vi "Station_NG Station.vi"(8 "error in (no error)":errorcluster, 11 "Main":T1={"Tite"="", "Base path"=path "", "Table"=[], "Stations"=[], "Shield Array"=[], "UPHs"=[], "VISA"={"VISA"="", "baud rate"=9600, "data bits"=8, "parity"=enum."None", "stop bits"=10, "flow control"=0}, "Path"={"roof"=path "", "Config"=path "", "Png"=path ""}, "Ctr"={"DB Dispaly"=refnum, "Error Table"=refnum, "Display"=refnum, "Login"=refnum, "Exit"=refnum, "FTT_Submit"=refnum}, "Login"={"User"="", "Grade"=""}, "information"={"cause"="", "Type"=enum."Inform", "code"=0, "Suroce"="", "Status"=FALSE}, "Local DB"={"Connstr"="", "Database"={"Constr"={"Driver"="", "Server"="", "User"="", "Pwd"="", "Database"=""}, "conn ref"=refnum, "State"=FALSE}}, "Remote DB"={"Connstr"="", "Database"={"Constr"={"Driver"="", "Server"="", "User"="", "Pwd"="", "Database"=""}, "conn ref"=refnum, "State"=FALSE}}, "FTT TV"="", "ExchangeTime"=0, "NVH"="", "EOL Path"=path ""} {"VISA"."flow control" items=["None", "XON/XOFF", "RTS/CTS", "XON/XOFF & RTS/CTS", "DTR/DSR", "XON/XOFF & DTR/DSR"]; "VISA"."stop bits" items=["1.0"=10, "1.5"=15, "2.0"=20]}) -> (0 "error out":errorcluster)   [LabVIEW 2014]
uses:
  Type'def/Online_Table.ctl
  <vilib>/addons/database/_DB Variant To Data/Database Variant To Data.xnode
  Simatic S7/Function/Read/Read Sigle Data/Read Sigle String.vi
  Simatic S7/Function/Read/Read Sigle Data/Read Sigle Word.vi
  Type'def/UPH Config.ctl
  VISA/Ctr/VISA Ctr.ctl
  Type'def/Main Ctr Ref.ctl
  Type'def/User Login.ctl
  Database/Ctr/Constr.ctl
  <vilib>/addons/database/Connection.llb/Conn ObjectReference.ctl
  <vilib>/addons/database/NI_Database_API.lvlib
  Database/Ctr/Conneect State.ctl
  Type'def/MainCtr.ctl
panel:
  in  "t":u16
  in  "s":bool
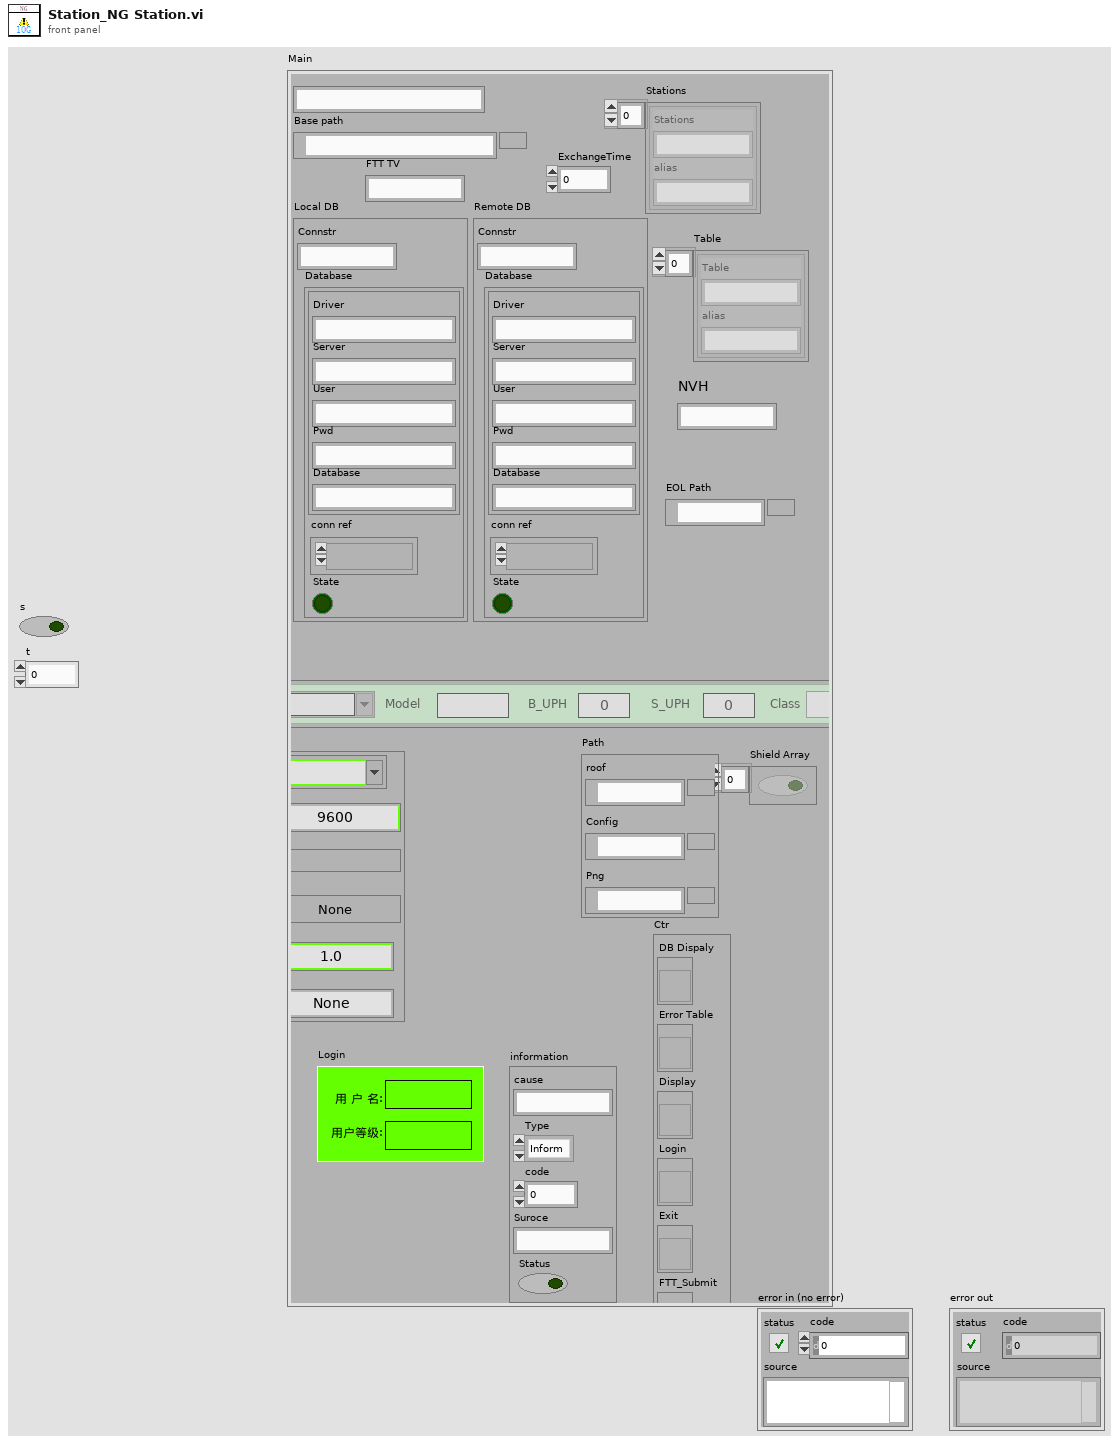
[diagram p1: front panel]
types:
  T1 = typedef "MainCtr.ctl" = cluster{"Tite":string, "Base path":path, "Table":cluster{"Table":string, "alias":string}[], "Stations":cluster{"Stations":string, "alias":string}[], "Shield Array":bool[], "UPHs":T2[], "VISA":T3, "Path":cluster{"roof":path, "Config":path, "Png":path}, "Ctr":T4, "Login":T5, "information":cluster{"cause":string, "Type":enum16{"Inform", "Warning", "Alarm"}, "code":i32, "Suroce":string, "Status":bool}, "Local DB":cluster{"Connstr":string, "Database":T6}, "Remote DB":cluster{"Connstr":string, "Database":T6}, "FTT TV":string, "ExchangeTime":i32, "NVH":string, "EOL Path":path}
  T2 = typedef "UPH Config.ctl" = cluster{"Line_No":string, "Model":string, "B_UPH ":i16, "S_UPH  ":i16, "Class":enum16{"Big", "Small"}}
  T3 = typedef "VISA Ctr.ctl" = cluster{"VISA":refnum<visa-resource-name>, "baud rate":u32, "data bits":u16, "parity":enum16{"None", "Odd", "Even", "Mark", "Space"}, "stop bits":u16, "flow control":u16}
  T4 = typedef "Main Ctr Ref.ctl" = cluster{"DB Dispaly":refnum<vi>, "Error Table":refnum<vi>, "Display":refnum<vi>, "Login":refnum<vi>, "Exit":refnum<vi>, "FTT_Submit":refnum<vi>}
  T5 = typedef "User Login.ctl" = cluster{"User":string, "Grade":string}
  T6 = typedef "Conneect State.ctl" = cluster{"Constr":T7, "conn ref":T8, "State":bool}
  T7 = typedef "Constr.ctl" = cluster{"Driver":string, "Server":string, "User":string, "Pwd":string, "Database":string}
  T8 = typedef "NI_Database_API.lvlib/Conn ObjectReference.ctl" = refnum<k1>
  T9 = cluster{"cause":string, "Type":enum16{"Inform", "Warning", "Alarm"}, "code":i32, "Suroce":string, "Status":bool}
  T10 = typedef "Online_Table.ctl" = cluster{"SN":string, "Frame":string, "Station":string, "Model":string, "Color":string, "OnTime":timestamp, "OutTime":timestamp, "Repaired":i32, "OnRepair":bool, "Pstate":string}
  T11 = cluster{"Main ":T1, "Online_Table":T10, "information":cluster{"cause":string, "Type":enum16{"Inform", "Warning", "Alarm"}, "code":i32, "Suroce":string, "Status":bool}, "Previous ":u16, "Station pos":i32[], "Pos":i32}
  T12 = typedef "FTT Display Type.ctl" = cluster{"Line.No":string, "Model":string, "Color":string, "UPH":dbl, "Plan":dbl, "Target Rate":dbl, "Target ":dbl, "Actual":dbl, "FTT":dbl, "FTT Rate":dbl, "Repaired":dbl, "Reject":dbl, "Ouline":dbl, "Line State":string}
  T13 = cluster{"Display":T12, "Class":enum16{"Big", "Small"}}
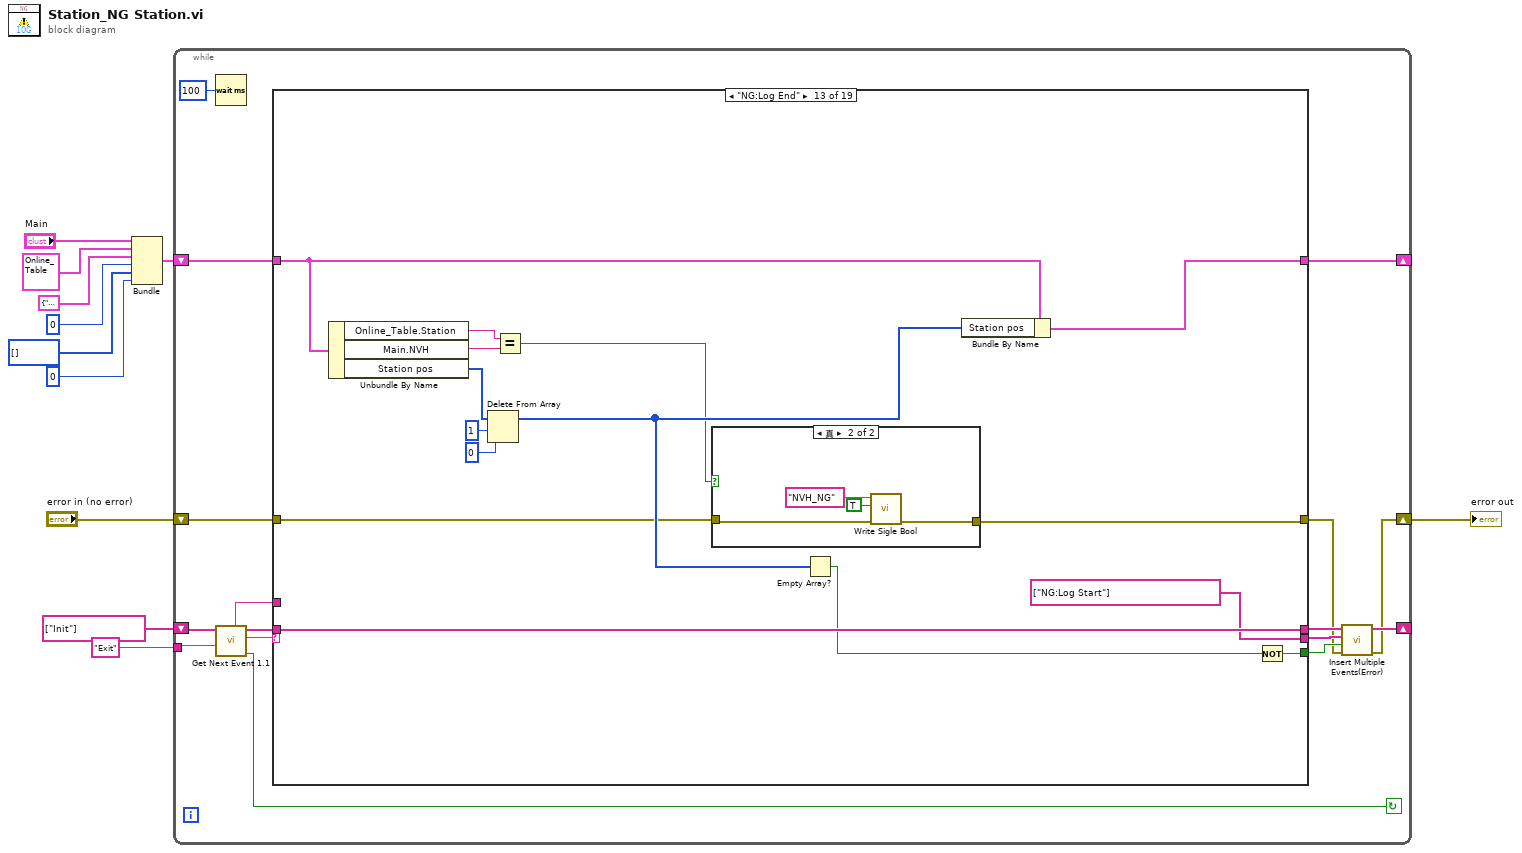
[diagram p0: block diagram]
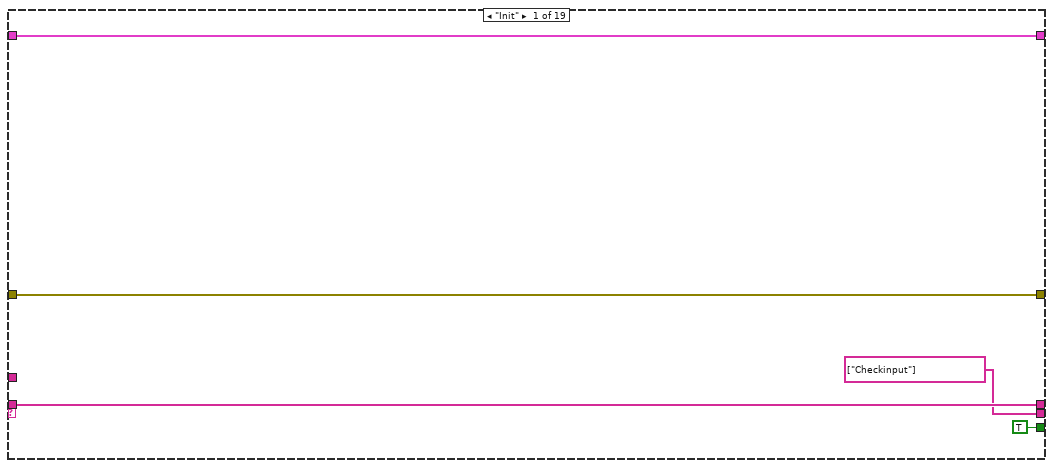
[diagram p2: hidden frame]
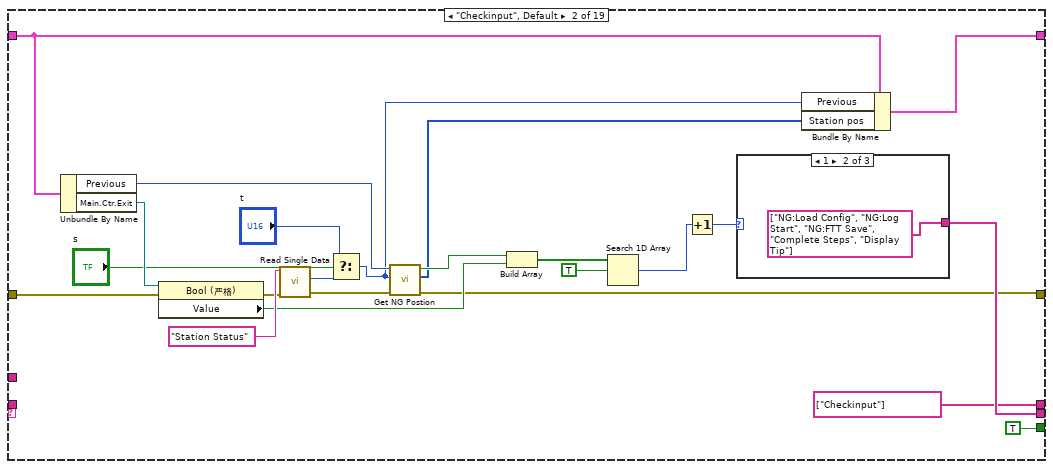
[diagram p3: hidden frame]
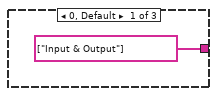
[diagram p4: hidden frame]
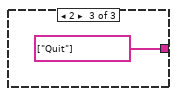
[diagram p5: hidden frame]
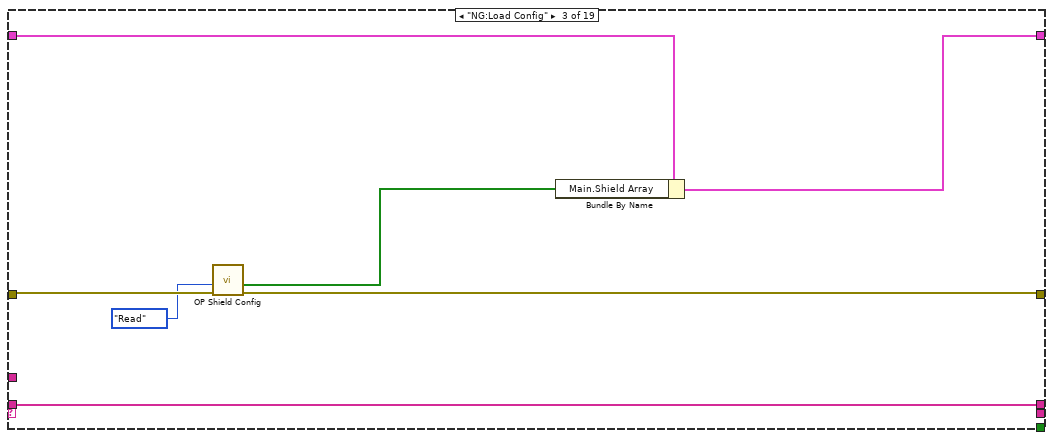
[diagram p6: hidden frame]
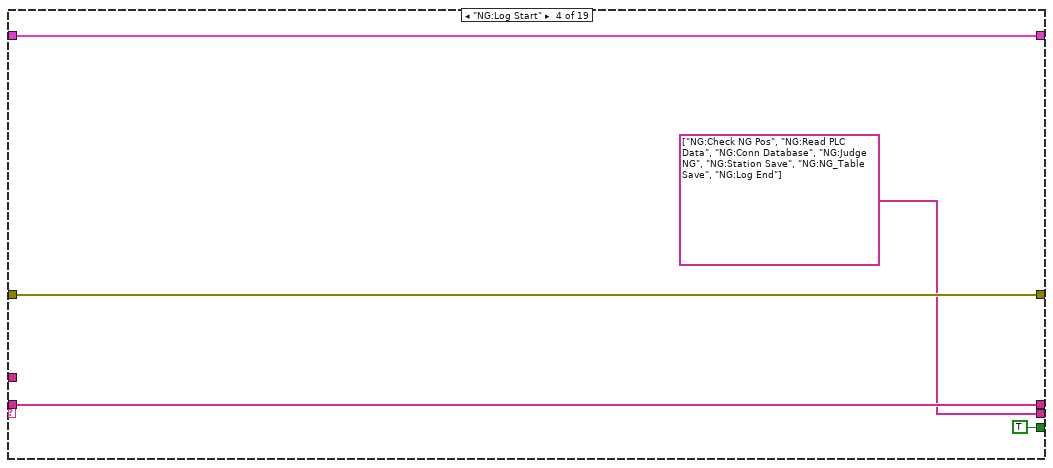
[diagram p7: hidden frame]
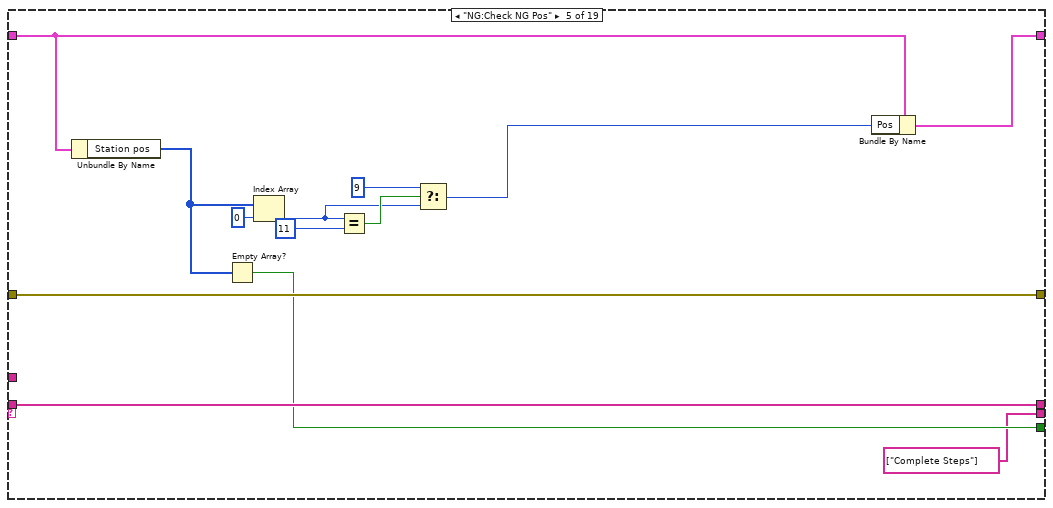
[diagram p8: hidden frame]
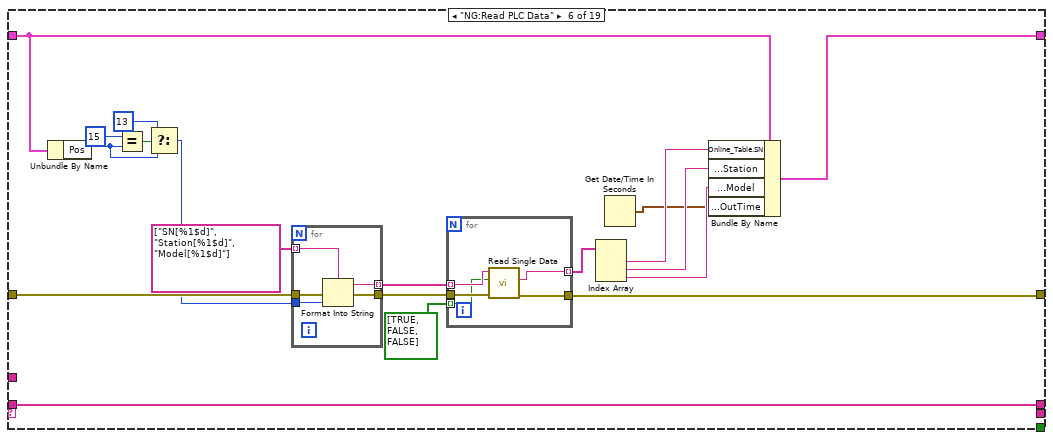
[diagram p9: hidden frame]
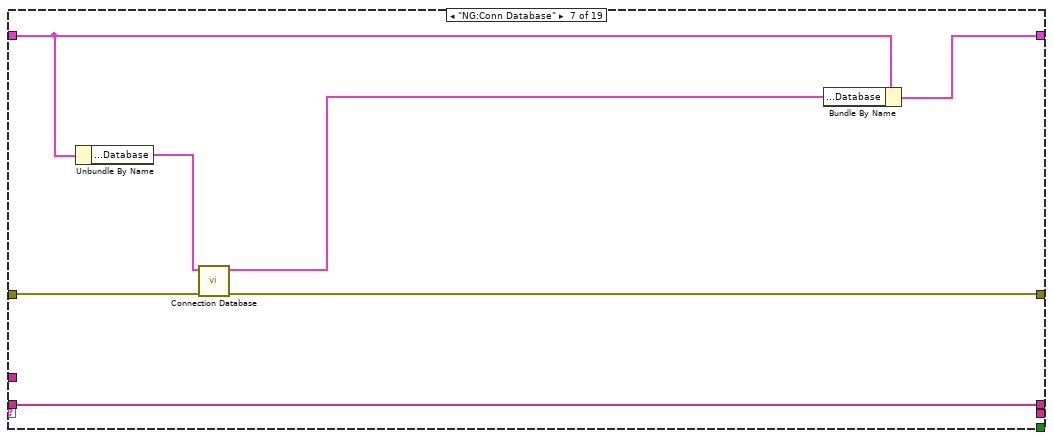
[diagram p10: hidden frame]
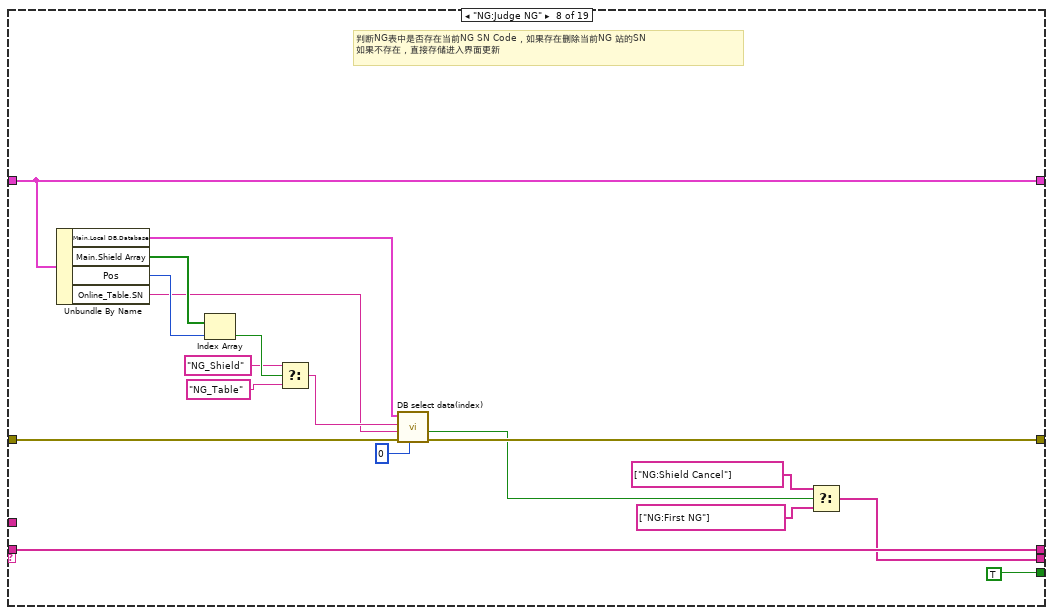
[diagram p11: hidden frame]
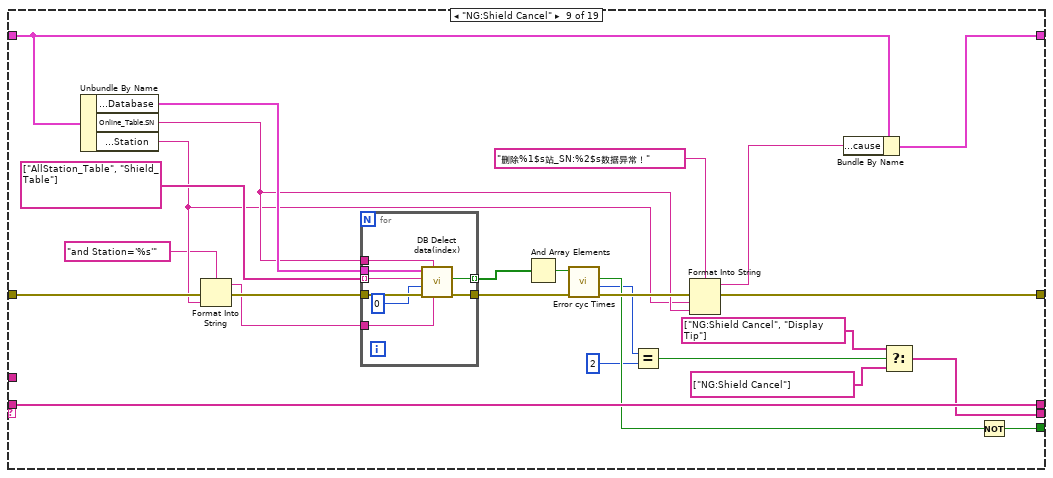
[diagram p12: hidden frame]
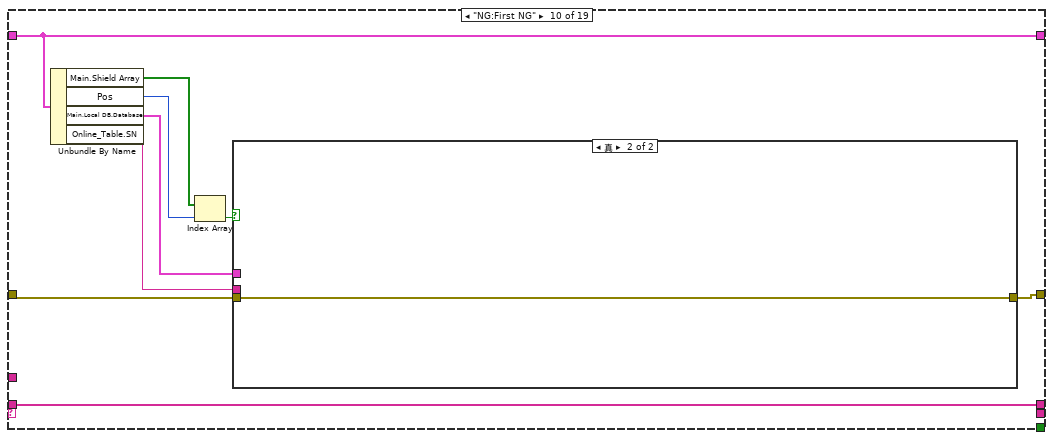
[diagram p13: hidden frame]
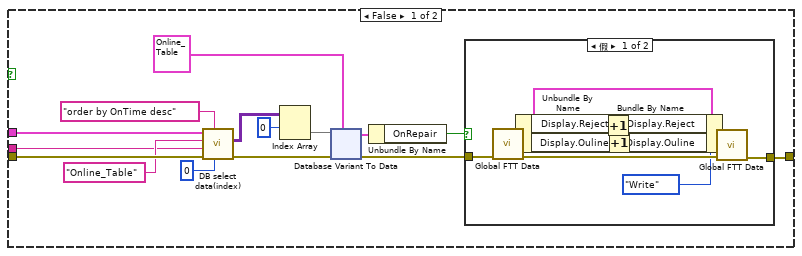
[diagram p14: hidden frame]
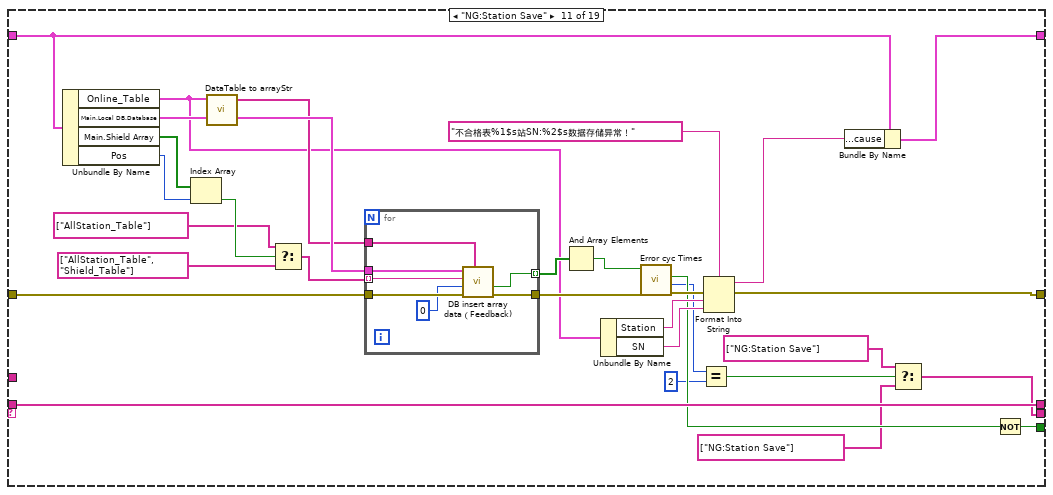
[diagram p16: hidden frame]
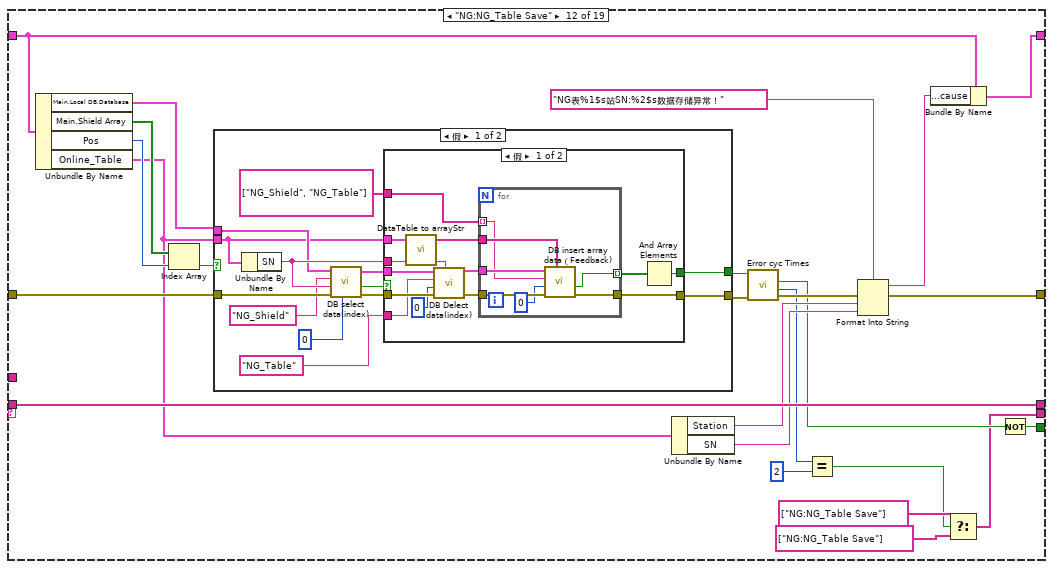
[diagram p17: hidden frame]
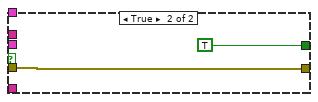
[diagram p18: hidden frame]
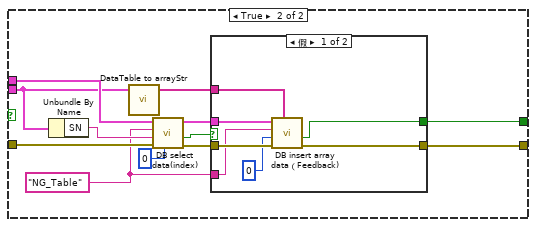
[diagram p19: hidden frame]
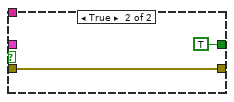
[diagram p20: hidden frame]
diagram:
  n1 = Bundle("Main"="Main", "Online_Table"=T10 {"SN"="", "Frame"="", "Station"="", "Model"="", "Color"="", "OnTime"=timestamp(0 s since 1904-01-01), "OutTime"=timestamp(0 s since 1904-01-01), "Repaired"=0, "OnRepair"=FALSE, "Pstate"=""}, "information"=T9 {"cause"="", "Type"=enum."Inform", "code"=0, "Suroce"="", "Status"=FALSE}, "Previous"=u16 0, "Station pos"=i32[] [], "Pos"=0) -> (w8:T11)  [unwired: 1 in]
  n2 = while {
    tunnel: "Exit" ("Exit Event") -> [w24]
    shift-right: [w20] -> _
    shift-left: string[] ["Init"] -> [w25]
    shift-right: [w13] -> w5
    shift-left: "error in (no error)" -> [w23]
    shift-right: [w16] -> _
    shift-left: w8 -> [w21]
    stop <- w26 continue-if-true
    n3 = Wait (ms)(milliseconds to wait=u32 100 ("等待时间（毫秒）")) -> ()  [unwired: 1 out]
    n4 = call "Get Next Event 1.1.vi"("Exit Event"=w24, "event queue in"=w25) -> ("Condition (Exit:F)"=w26:bool, "next event"=w27:string, "event queue out"=w22:string[], "Previous Event"=w15:string)  [unwired: 6 in]
    n5 = case shown="\"NG:Log End\"" w27 {
      tunnel: w23 -> [w30 w54 w64 w68 w83 w99 w119 w131 w160 w178 w572 w606 w668 w708 w764 w771 w776 w782 w784]
      tunnel: w22 -> [w32 _ w65 w69 w82 w102 w116 w126 w163 w180 w568 w604 w680 w712 w765 w768 w775 w778 w787]
      tunnel: w21 -> [w31 w39 w60 w70 w79 w100 w115 w137 w154 w179 w557 w588 w676 w691 w760 w772 w777 w780 w791]
      tunnel: [w30 w41 w63 w68 w83 w98 w117 w125 w149 w172 w558 w591 w666 w700 w762 w769 w776 w781 w792] -> w14
      tunnel: [w32 string[] ["Checkinput"] w65 w69 w82 w102 w116 w126 w163 w180 w568 w604 w680 w712 w765 w768 w775 w778 w787] -> w19
      tunnel: [TRUE ("Insert all? (T)") TRUE ("Insert all? (T)") _ TRUE ("Insert all? (T)") w81 _ _ TRUE w147 _ w555 w593 w673 w698 _ w767 TRUE ("Insert all? (T)") _ TRUE ("Insert all? (T)")] -> w18
      tunnel: [string[] ["Checkinput"] w46 _ string[] ["NG:Check NG Pos", "NG:Read PLC Data", "NG:Conn Database", "NG:Judge NG", "NG:Station Save", "NG:NG_Table Save", "NG:Log End"] string[] ["Complete Steps"] _ _ w120 w143 _ w549 w590 string[] ["NG:Log Start"] w693 _ string[] ["Quit"] string[] ["Exit"] _ string[] ["Checkinput"]] -> w17
      tunnel: [w31 w38 w59 w70 w78 w101 w114 w137 w153 w179 w556 w587 w675 w690 w759 w772 w777 w780 w791] -> w16
      tunnel: w15 -> [_ _ _ _ _ _ _ _ _ _ _ _ _ _ _ _ _ _ _]
      frame "Init" {
      }
      frame "Checkinput", Default {
        n6 = Unbundle By Name(w39) -> ("Previous"=w43:u16, "Main.Ctr.Exit"=w55:refnum<vi>)
        n7 = property class="Bool (严格)"(reference=w55, error in=w54) -> (error out=w45:errorcluster, "Value"=w52:bool)  [unwired: 1 out]
        n8 = call-poly "Read Single Data.vi"("error in (no error)"=w45, "Tags"="Station Status") -> ("error out"=w44:errorcluster, "Data Byte"=w36:u16)  [unwired: 7 in, 1 out]
        n9 = Select(t="t", s="s", f=w36) -> (s? t:f=w35:u16)
        n10 = call "Get NG Postion.vi"("error in (no error)"=w44, "Current"=w35, "Previous"=w43) -> ("error out"=w41:errorcluster, "Station pos"=w40:i32[], "Status"=w42:bool)  [unwired: 6 in]
        n11 = Build Array(w42, w52) -> (w51:bool[])
        n12 = Search 1D Array(1D array=w51, element=TRUE) -> (index of element=w49:i32)  [unwired: 1 in]
        n13 = Increment(x=w49) -> (x+1=w47:i32)
        n14 = case shown="1" w47 {
          tunnel: [string[] ["Input & Output"] string[] ["NG:Load Config", "NG:Log Start", "NG:FTT Save", "Complete Steps", "Display Tip"] string[] ["Quit"]] -> w46
          frame 0, Default {
          }
          frame 1 {
          }
          frame 2 {
          }
        }
        n15 = Bundle By Name(cluster=w39, "Previous"=w35, "Station pos"=w40) -> (w38:T11)
      }
      frame "NG:Load Config" {
        n16 = call "OP Shield Config.vi"("error in (no error)"=w64, "Enum"=enum16{"init", "Read", "Write"}."Read") -> ("error out"=w63:errorcluster, "subarray"=w61:bool[])  [unwired: 6 in, 2 out]
        n17 = Bundle By Name(cluster=w60, "Main.Shield Array"=w61) -> (w59:T11)
      }
      frame "NG:Log Start" {
      }
      frame "NG:Check NG Pos" {
        n18 = Unbundle By Name(w79) -> ("Station pos"=w77:i32[])
        n19 = Empty Array?(array=w77) -> (empty?=w81:bool)
        n20 = Index Array(array=w77, index=0) -> (element=w73:i32)
        n21 = Equal?(x=w73, y=11) -> (x = y?=w74:bool)
        n22 = Select(t=9, s=w74, f=w73) -> (s? t:f=w71:i32)
        n23 = Bundle By Name(cluster=w79, "Pos"=w71) -> (w78:T11)
      }
      frame "NG:Read PLC Data" {
        n24 = Unbundle By Name(w100) -> ("Pos"=w86:i32)
        n25 = Equal?(x=15, y=w86) -> (x = y?=w87:bool)
        n26 = Select(t=13, s=w87, f=w86) -> (s? t:f=w84:i32)
        n27 = for {
          tunnel: w99 -> [w107]
          tunnel: w84 -> [w106]
          tunnel: string[] ["SN[%1$d]", "Station[%1$d]", "Model[%1$d]"] -> [w105] mode=indexing
          tunnel: [w104] -> w93
          tunnel: [w103] -> w92 mode=indexing
          n28 = Format Into String(format string=w105, error in=w107, w106) -> (resulting string=w103:string, error out=w104:errorcluster)  [unwired: 1 in]
        }
        n29 = for {
          tunnel: [w112] -> w98
          tunnel: [w111] -> w97 mode=indexing
          tunnel: w93 -> [w110]
          tunnel: w92 -> [w109] mode=indexing
          tunnel: bool[] [TRUE, FALSE, FALSE] -> [w108] mode=indexing
          n30 = call-poly "Read Single Data.vi"("error in (no error)"=w110, "Char/Str"=w108, "Tags"=w109) -> ("error out"=w112:errorcluster, "Data Byte"=w111:string)  [unwired: 6 in, 1 out]
        }
        n31 = Index Array(array=w97) -> (element #1=w96:string, element #2=w95:string, element #3=w91:string)  [unwired: 3 in]
        n32 = Get Date/Time In Seconds() -> (seconds since 1Jan1904=w90:timestamp)
        n33 = Bundle By Name(cluster=w100, "Online_Table.SN"=w96, "Online_Table.Station"=w95, "Online_Table.Model"=w91, "Online_Table.OutTime"=w90) -> (w101:T11)
      }
      frame "NG:Conn Database" {
        n34 = Unbundle By Name(w115) -> ("Main.Local DB.Database"=w118:T6)
        n35 = call "Connection Database.vi"("error in (no error)"=w119, "Connncet State"=w118) -> ("error out"=w117:errorcluster, "Connncet State out"=w113:T6)  [unwired: 8 in]
        n36 = Bundle By Name(cluster=w115, "Main.Local DB.Database"=w113) -> (w114:T11)
      }
      frame "NG:Judge NG" {
        # "判断NG表中是否存在当前NG SN Code，如果存在删除当前NG 站的SN\n如果不存在，直接存储进入界面更新"
        n37 = Unbundle By Name(w137) -> ("Main.Local DB.Database"=w130:T6, "Main.Shield Array"=w136:bool[], "Pos"=w135:i32, "Online_Table.SN"=w128:string)
        n38 = Index Array(array=w136, index=w135) -> (element=w134:bool)
        n39 = Select(t="NG_Shield", s=w134, f="NG_Table") -> (s? t:f=w129:string)
        n40 = call "DB select data(index).vi"("index"=0, "error in (no error)"=w131, "Code"=w128, "Tabe"=w129, "Connncet State"=w130) -> ("error out"=w125:errorcluster, "state"=w123:bool)  [unwired: 3 in, 2 out]
        n41 = Select(t=string[] ["NG:Shield Cancel"], s=w123, f=string[] ["NG:First NG"]) -> (s? t:f=w120:string[])
      }
      frame "NG:Shield Cancel" {
        n42 = Unbundle By Name(w154) -> ("Main.Local DB.Database"=w162:T6, "Online_Table.SN"=w150:string, "Online_Table.Station"=w139:string)
        n43 = Format Into String(format string="and Station='%s'", error in=w160, w139) -> (resulting string=w158:string, error out=w159:errorcluster)  [unwired: 1 in]
        n44 = for {
          tunnel: w159 -> [w171]
          tunnel: w162 -> [w170]
          tunnel: string[] ["AllStation_Table", "Shield_Table"] -> [w169] mode=indexing
          tunnel: w150 -> [w167]
          tunnel: w158 -> [w166]
          tunnel: [w165] -> w156
          tunnel: [w164] -> w157 mode=indexing
          n45 = call "DB Delect data(index).vi"("Condtion"=w166, "code"=w167, "error in (no error)"=w171, "index"=0, "table"=w169, "Connncet State"=w170) -> ("error out"=w165:errorcluster, "Boolean"=w164:bool)  [unwired: 3 in, 1 out]
        }
        n46 = And Array Elements(Boolean array=w157) -> (logical AND=w155:bool)
        n47 = call "Error cyc Times.vi"("error in (no error)"=w156, "Status in"=w155) -> ("error out"=w152:errorcluster, "Numeric"=w141:i32, "Cys Status"=w146:bool)  [unwired: 6 in, 1 out]
        n48 = Equal?(x=w141, y=2) -> (x = y?=w140:bool)
        n49 = Format Into String(format string="删除%1$s站_SN:%2$s数据异常！", error in=w152, w139, w150) -> (resulting string=w148:string, error out=w149:errorcluster)  [unwired: 1 in]
        n50 = Bundle By Name(cluster=w154, "information.cause"=w148) -> (w153:T11)
        n51 = Select(t=string[] ["NG:Shield Cancel", "Display Tip"], s=w140, f=string[] ["NG:Shield Cancel"]) -> (s? t:f=w143:string[])
        n52 = Not(x=w146) -> (.not. x?=w147:bool)
      }
      frame "NG:First NG" {
        n53 = Unbundle By Name(w179) -> ("Main.Shield Array"=w175:bool[], "Pos"=w174:i32, "Main.Local DB.Database"=w177:T6, "Online_Table.SN"=w176:string)
        n54 = Index Array(array=w175, index=w174) -> (element=w173:bool)
        n55 = case shown="真" w173 {
          tunnel: w178 -> [w195 w547]
          tunnel: w177 -> [w194 _]
          tunnel: w176 -> [w192 _]
          tunnel: [w181 w547] -> w172
          frame False {
            n56 = call "DB select data(index).vi"("index"=0, "Condtion"="order by OnTime desc", "error in (no error)"=w195, "Code"=w192, "Tabe"="Online_Table", "Connncet State"=w194) -> ("error out"=w187:errorcluster, "data"=w189:variant[][])  [unwired: 2 in, 2 out]
            n57 = Index Array(array=w189, index (row)=0) -> (element=w186:variant[])  [unwired: 1 in]
            n58 = xnode "Database Variant To Data"("database variant"=w186, "error in (no error)"=w187, "type"=T10 {"SN"="", "Frame"="", "Station"="", "Model"="", "Color"="", "OnTime"=timestamp(0 s since 1904-01-01), "OutTime"=timestamp(0 s since 1904-01-01), "Repaired"=0, "OnRepair"=FALSE, "Pstate"=""} ("Online_Table")) -> ("data"=w184:T10, "error out"=w182:errorcluster)
            n59 = Unbundle By Name(w184) -> ("OnRepair"=w183:bool)
            n60 = case shown="假" w183 {
              tunnel: w182 -> [w205 w206]
              tunnel: [w196 w206] -> w181
              frame False {
                n61 = call "Global FTT Data.vi"("error in (no error)"=w205) -> ("error out"=w199:errorcluster, "Cluster"=w202:T13)  [unwired: 9 in]
                n62 = Unbundle By Name(w202) -> ("Display.Reject"=w204:dbl, "Display.Ouline"=w203:dbl)
                n63 = Increment(x=w204) -> (x+1=w201:dbl)
                n64 = Increment(x=w203) -> (x+1=w200:dbl)
                n65 = Bundle By Name(cluster=w202, "Display.Reject"=w201, "Display.Ouline"=w200) -> (w198:T13)
                n66 = call "Global FTT Data.vi"("error in (no error)"=w199, "Mode"=enum16{"Read", "Write"}."Write", "Display"=w198) -> ("error out"=w196:errorcluster)  [unwired: 7 in, 1 out]
              }
              frame True {
              }
            }
          }
          frame True {
          }
        }
      }
      frame "NG:Station Save" {
        n67 = Unbundle By Name(w557) -> ("Online_Table"=w562:T10, "Main.Local DB.Database"=w571:T6, "Main.Shield Array"=w577:bool[], "Pos"=w576:i32)
        n68 = Index Array(array=w577, index=w576) -> (element=w575:bool)
        n69 = call "DataTable to arrayStr.vi"("Online_Table"=w562) -> ("appended array"=w569:string[])  [unwired: 4 in]
        n70 = Select(t=string[] ["AllStation_Table"], s=w575, f=string[] ["AllStation_Table", "Shield_Table"]) -> (s? t:f=w570:string[])
        n71 = for {
          tunnel: w572 -> [w584]
          tunnel: w571 -> [w583]
          tunnel: w570 -> [w582] mode=indexing
          tunnel: w569 -> [w580]
          tunnel: [w579] -> w566
          tunnel: [w578] -> w567 mode=indexing
          n72 = call "DB insert array data（Feedback).vi"("Data"=w580, "error in (no error)"=w584, "index"=0, "table"=w582, "Connncet State"=w583) -> ("error out"=w579:errorcluster, "state"=w578:bool)  [unwired: 4 in, 1 out]
        }
        n73 = And Array Elements(Boolean array=w567) -> (logical AND=w565:bool)
        n74 = Unbundle By Name(w562) -> ("Station"=w561:string, "SN"=w560:string)
        n75 = call "Error cyc Times.vi"("error in (no error)"=w566, "Status in"=w565) -> ("error out"=w564:errorcluster, "Numeric"=w553:i32, "Cys Status"=w554:bool)  [unwired: 6 in, 1 out]
        n76 = Equal?(x=w553, y=2) -> (x = y?=w551:bool)
        n77 = Format Into String(format string="不合格表%1$s站SN:%2$s数据存储异常！", error in=w564, w561, w560) -> (resulting string=w559:string, error out=w558:errorcluster)  [unwired: 1 in]
        n78 = Bundle By Name(cluster=w557, "information.cause"=w559) -> (w556:T11)
        n79 = Select(t=string[] ["NG:Station Save"], s=w551, f=string[] ["NG:Station Save"]) -> (s? t:f=w549:string[])
        n80 = Not(x=w554) -> (.not. x?=w555:bool)
      }
      frame "NG:NG_Table Save" {
        n81 = Unbundle By Name(w588) -> ("Main.Local DB.Database"=w605:T6, "Main.Shield Array"=w609:bool[], "Pos"=w608:i32, "Online_Table"=w596:T10)
        n82 = Index Array(array=w609, index=w608) -> (element=w607:bool)
        n83 = case shown="假" w607 {
          tunnel: w606 -> [w622 w656]
          tunnel: w605 -> [w611 w655]
          tunnel: w596 -> [w610 w648]
          tunnel: [w618 w651] -> w597
          tunnel: [w617 w645] -> w595
          frame False {
            n84 = Unbundle By Name(w610) -> ("SN"=w615:string)
            n85 = call "DB select data(index).vi"("index"=0, "error in (no error)"=w622, "Code"=w615, "Tabe"="NG_Shield", "Connncet State"=w611) -> ("error out"=w620:errorcluster, "state"=w619:bool, "Connncet State out"=w616:T6)  [unwired: 3 in, 1 out]
            n86 = case shown="假" w619 {
              tunnel: w620 -> [w635 w644]
              tunnel: [w625 w644] -> w618
              tunnel: [w623 TRUE] -> w617
              tunnel: w616 -> [w634 _]
              tunnel: w615 -> [w633 _]
              tunnel: "NG_Table" -> [w632 _]
              tunnel: string[] ["NG_Shield", "NG_Table"] -> [w626 _]
              tunnel: w610 -> [w629 _]
              frame False {
                n87 = call "DataTable to arrayStr.vi"("Online_Table"=w629) -> ("appended array"=w628:string[])  [unwired: 4 in]
                n88 = call "DB Delect data(index).vi"("code"=w633, "error in (no error)"=w635, "index"=0, "table"=w632, "Connncet State"=w634) -> ("error out"=w630:errorcluster, "Connncet State out"=w627:T6)  [unwired: 4 in, 1 out]
                n89 = for {
                  tunnel: w630 -> [w642]
                  tunnel: w628 -> [w641]
                  tunnel: w627 -> [w640]
                  tunnel: w626 -> [w638] mode=indexing
                  tunnel: [w637] -> w625
                  tunnel: [w636] -> w624 mode=indexing
                  n90 = call "DB insert array data（Feedback).vi"("Data"=w641, "error in (no error)"=w642, "index"=0, "table"=w638, "Connncet State"=w640) -> ("error out"=w637:errorcluster, "state"=w636:bool)  [unwired: 4 in, 1 out]
                }
                n91 = And Array Elements(Boolean array=w624) -> (logical AND=w623:bool)
              }
              frame True {
              }
            }
          }
          frame True {
            w646 = "NG_Table"
            n92 = Unbundle By Name(w648) -> ("SN"=w649:string)
            n93 = call "DataTable to arrayStr.vi"("Online_Table"=w648) -> ("appended array"=w647:string[])  [unwired: 4 in]
            n94 = call "DB select data(index).vi"("index"=0, "error in (no error)"=w656, "Code"=w649, "Tabe"=w646, "Connncet State"=w655) -> ("error out"=w653:errorcluster, "state"=w652:bool, "Connncet State out"=w650:T6)  [unwired: 3 in, 1 out]
            n95 = case shown="假" w652 {
              tunnel: w653 -> [w663 w665]
              tunnel: [w658 w665] -> w651
              tunnel: w650 -> [w662 _]
              tunnel: w647 -> [w661 _]
              tunnel: w646 -> [w660 _]
              tunnel: [w657 TRUE ("state")] -> w645
              frame False {
                n96 = call "DB insert array data（Feedback).vi"("Data"=w661, "error in (no error)"=w663, "index"=0, "table"=w660, "Connncet State"=w662) -> ("error out"=w658:errorcluster, "state"=w657:bool)  [unwired: 4 in, 1 out]
              }
              frame True {
              }
            }
          }
        }
        n97 = Unbundle By Name(w596) -> ("Station"=w599:string, "SN"=w600:string)
        n98 = call "Error cyc Times.vi"("error in (no error)"=w597, "Status in"=w595) -> ("error out"=w598:errorcluster, "Numeric"=w594:i32, "Cys Status"=w592:bool)  [unwired: 6 in, 1 out]
        n99 = Equal?(x=w594, y=2) -> (x = y?=w589:bool)
        n100 = Format Into String(format string="NG表%1$s站SN:%2$s数据存储异常！", error in=w598, w599, w600) -> (resulting string=w586:string, error out=w591:errorcluster)  [unwired: 1 in]
        n101 = Bundle By Name(cluster=w588, "information.cause"=w586) -> (w587:T11)
        n102 = Select(t=string[] ["NG:NG_Table Save"], s=w589, f=string[] ["NG:NG_Table Save"]) -> (s? t:f=w590:string[])
        n103 = Not(x=w592) -> (.not. x?=w593:bool)
      }
      frame "NG:Log End" {
        n104 = Unbundle By Name(w676) -> ("Online_Table.Station"=w669:string, "Main.NVH"=w670:string, "Station pos"=w679:i32[])
        n105 = Delete From Array(array=w679, length=1, index=0) -> (array with subset deleted=w674:i32[])  [unwired: 1 out]
        n106 = Equal?(x=w669, y=w670) -> (x = y?=w667:bool)
        n107 = case shown="真" w667 {
          tunnel: w668 -> [w681 w685]
          tunnel: [w681 w684] -> w666
          frame False {
          }
          frame True {
            n108 = call "Write Sigle Bool.vi"("error in (no error)"=w685, "Data"=TRUE, "Tags"="NVH_NG") -> ("error out"=w684:errorcluster)  [unwired: 6 in, 2 out]
          }
        }
        n109 = Empty Array?(array=w674) -> (empty?=w672:bool)
        n110 = Bundle By Name(cluster=w676, "Station pos"=w674) -> (w675:T11)
        n111 = Not(x=w672) -> (.not. x?=w673:bool)
      }
      frame "NG:FTT Save" {
        n112 = Unbundle By Name(w691) -> ("Main.Local DB.Database"=w709:T6, "Online_Table.Station"=w702:string, "Online_Table.SN"=w701:string)
        n113 = call "Global FTT Data.vi"("error in (no error)"=w708) -> ("error out"=w707:errorcluster, "Cluster"=w687:T13)  [unwired: 9 in]
        n114 = Unbundle By Name(w687) -> ("Display.Line.No"=w706:string)
        n115 = Unbundle By Name(w687) -> ("Display"=w686:T12)
        n116 = First Call?() -> (First Call?: T/F=w711:bool)
        n117 = case shown="真" w711 {
          tunnel: w707 -> [w722 w733]
          tunnel: "[FTT_Clinet].[dbo].[FTT1_ Write]" -> [w720 w728]
          tunnel: w709 -> [w721 w732]
          tunnel: w706 -> [w719 w723]
          tunnel: w686 -> [w714 w724]
          tunnel: [w716 w726] -> w705
          tunnel: [w715 w725] -> w699
          frame False {
            n118 = To Variant(anything=w714) -> (Variant=w713:variant)
            n119 = call "DB Update Data(Feedback).vi"("Pos"=cluster{"index":i32, "Len":i32} {"index"=0, "Len"=14}, "Sel index"=0, "data"=w713, "error in (no error)"=w722, "Code"=w719, "table"=w720, "Connncet State"=w721) -> ("error out"=w716:errorcluster, "State"=w715:bool)  [unwired: 2 in, 1 out]
          }
          frame True {
            n120 = call "ftt array.vi"("Display"=w724) -> ("appended array"=w727:string[])  [unwired: 4 in]
            n121 = call "DB select data(index).vi"("error in (no error)"=w733, "Code"=w723, "Tabe"=w728, "Connncet State"=w732) -> ("error out"=w731:errorcluster, "state"=w730:bool, "Connncet State out"=w729:T6)  [unwired: 4 in, 1 out]
            n122 = case shown="真" w730 {
              tunnel: w731 -> [w741 w749]
              tunnel: w729 -> [w740 w744]
              tunnel: w728 -> [w739 w743]
              tunnel: w727 -> [w737 _]
              tunnel: [w736 w748] -> w726
              tunnel: [w735 w747] -> _
              tunnel: [w734 w746] -> w725
              tunnel: w724 -> [_ w745]
              tunnel: w723 -> [_ w742]
              frame False {
                n123 = call "DB insert array data（Feedback).vi"("Data"=w737, "error in (no error)"=w741, "index"=0, "table"=w739, "Connncet State"=w740) -> ("error out"=w736:errorcluster, "state"=w734:bool, "Connncet State out"=w735:T6)  [unwired: 4 in]
              }
              frame True {
                n124 = call "DB Update Data(Feedback).vi"("Pos"=cluster{"index":i32, "Len":i32} {"index"=0, "Len"=14}, "Sel index"=0, "data"=w745, "error in (no error)"=w749, "Code"=w742, "table"=w743, "Connncet State"=w744) -> ("error out"=w748:errorcluster, "State"=w746:bool, "Connncet State out"=w747:T6)  [unwired: 2 in]
              }
            }
          }
        }
        n125 = call "Error cyc Times.vi"("error in (no error)"=w705, "Status in"=w699) -> ("error out"=w704:errorcluster, "Numeric"=w696:i32, "Cys Status"=w697:bool)  [unwired: 6 in, 1 out]
        n126 = Equal?(x=w696, y=2) -> (x = y?=w694:bool)
        n127 = Format Into String(format string="%1$s_SN:%2$s的FTT_Write表数据记录异常！", error in=w704, w702, w701) -> (resulting string=w692:string, error out=w700:errorcluster)  [unwired: 1 in]
        n128 = Bundle By Name(cluster=w691, "information.cause"=w692) -> (w690:T11)
        n129 = Select(t=string[] ["NG:FTT Save", "Display Tip"], s=w694, f=string[] ["NG:FTT Save"]) -> (s? t:f=w693:string[])
        n130 = Not(x=w697) -> (.not. x?=w698:bool)
      }
      frame "Complete Steps" {
        n131 = Unbundle By Name(w760) -> ("Online_Table.Station"=w754:string, "Online_Table.SN"=w753:string, "Main.Local DB.Database"=w763:T6)
        n132 = call "Disconncetion DB.vi"("error in (no error)"=w764, "Connncet State"=w763) -> ("error out"=w762:errorcluster, "Connect State"=w761:T6)  [unwired: 8 in]
        n133 = Concatenate Strings(w754, "SN:" ("string"), w753, "NG件数据记录完成" ("string")) -> (w756:string)
        n134 = Bundle By Name(cluster=w760, "Main.Local DB.Database"=w761, "information.cause"=w756, "Online_Table"=T10 {"SN"="", "Frame"="", "Station"="", "Model"="", "Color"="", "OnTime"=timestamp(0 s since 1904-01-01), "OutTime"=timestamp(0 s since 1904-01-01), "Repaired"=0, "OnRepair"=FALSE, "Pstate"=""}, "information.Status"=FALSE) -> (w759:T11)
      }
      frame "Input & Output" {
        n135 = Unbundle By Name(w772) -> ("Main.Ctr.Exit"=w770:refnum<vi>)
        n136 = property class="Bool (严格)"(reference=w770, error in=w771) -> (error out=w769:errorcluster, "Value"=w767:bool)  [unwired: 1 out]
      }
      frame "Quit" {
        # "软硬件关闭"
      }
      frame "Display Tip" {
        n137 = Unbundle By Name(w780) -> ("information"=w779:T9)
        n138 = call "Log info.vi"("error in (no error)"=w782, "information"=w779) -> ("error out"=w781:errorcluster)  [unwired: 8 in, 1 out]
      }
      frame "Error Log" {
        n139 = Unbundle By Name(w791) -> ("information"=w790:T9)
        n140 = Unbundle By Name(w784) -> ("source"=w783:string)
        n141 = Bundle By Name(cluster=w790, "Suroce"=w783, "Status"=TRUE) -> (w789:T9)
        n142 = call "Log info.vi"("error in (no error)"=w784, "information"=w789) -> ("error out"=w793:errorcluster)  [unwired: 8 in, 1 out]
        n143 = call <vilib>:"Clear Errors.vi"("error in (no error)"=w793) -> ("error out"=w792:errorcluster)  [unwired: 5 in, 1 out]
      }
    }
    n144 = call "Insert Multiple Events(Error).vi"("error in (no error)"=w14, "Insert all? (T)"=w18, "Events to Insert"=w17, "Event queue in"=w19) -> ("error out"=w13:errorcluster, "Event queue out"=w20:string[])  [unwired: 6 in]
  }
  "error out" <- w5
